vi "Read String Parameters from string.vi"(7 "String":string) -> (0 "error in (no error)":errorcluster, 3 "Parameters - string":T1[](array[typedef]))   [LabVIEW 2020, in "TALOS.lvlib" / "Run Utilities.lvlib" / "Optimiser Cell.lvclass"]
uses:
  Optimiser Cell.lvclass
  Optimise parameter - string.ctl
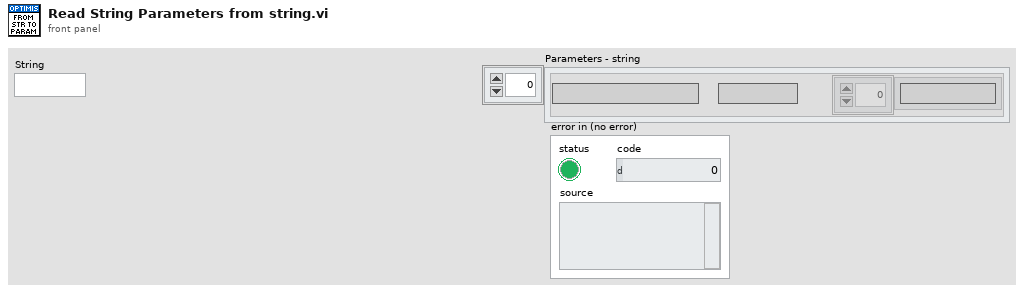
[diagram p1: front panel]
types:
  T1 = typedef "TALOS.lvlib/Run Utilities.lvlib/Optimiser Cell.lvclass/Optimise parameter - string.ctl" = cluster{"Name":string, "Start value":string, "Options":string[]}
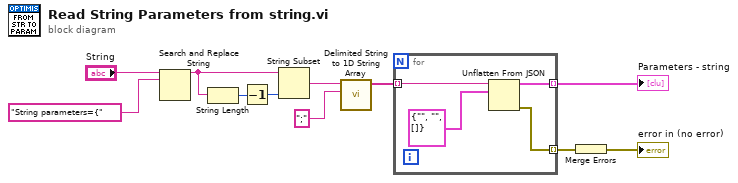
[diagram p0: block diagram]
diagram:
  n1 = Search and Replace String(input string="String", search string="String parameters={") -> (result string=w9:string)  [unwired: 6 in, 3 out]
  n2 = String Length(string=w9) -> (length=w8:i32)
  n3 = Decrement(x=w8) -> (x-1=w7:i32)
  n4 = String Subset(string=w9, length (rest)=w7) -> (substring=w6:string)  [unwired: 1 in]
  n5 = call <vilib>:"Delimited String to 1D String Array.vi"("delimiter"=";", "delimited string"=w6) -> ("string array"=w4:string[])  [unwired: 9 in]
  n6 = for {
    tunnel: [w14] -> w3 mode=indexing
    tunnel: [w13] -> w2 mode=indexing
    tunnel: w4 -> [w12] mode=indexing
    n7 = Unflatten From JSON(JSON string=w12, type and defaults=T1 {"Name"="", "Start value"="", "Options"=[]} ("input cluster 2")) -> (value=w14:T1, error out=w13:errorcluster)  [unwired: 5 in]
  }
  "Parameters - string" <- w3
  n8 = Merge Errors(w2) -> (→"error in (no error)":errorcluster)
